vi "Taller3.vi"(10 "U_OUT":dbl min=0.0 max=1.0 step=0.01, 11 "U_IN":dbl min=0.0 max=1.0 step=0.01) -> (0 "Numeric":dbl, 1 "Tank":dbl(slide) scale=0.0..3.3)   [LabVIEW 2024]
panel:
  in  "?":enum16{""}(ring)
  in  "Stop Button":bool
  in  "Alpha":dbl
  in  "A":dbl
  in  "K_OUT":dbl
  in  "DT":dbl
  in  "H_T":dbl
  in  "K_IN":dbl
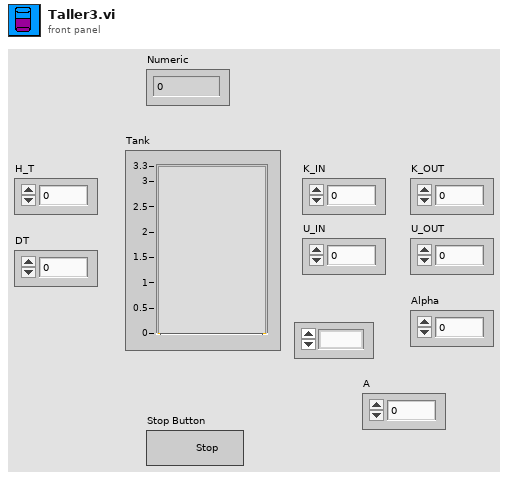
[diagram p1: front panel]
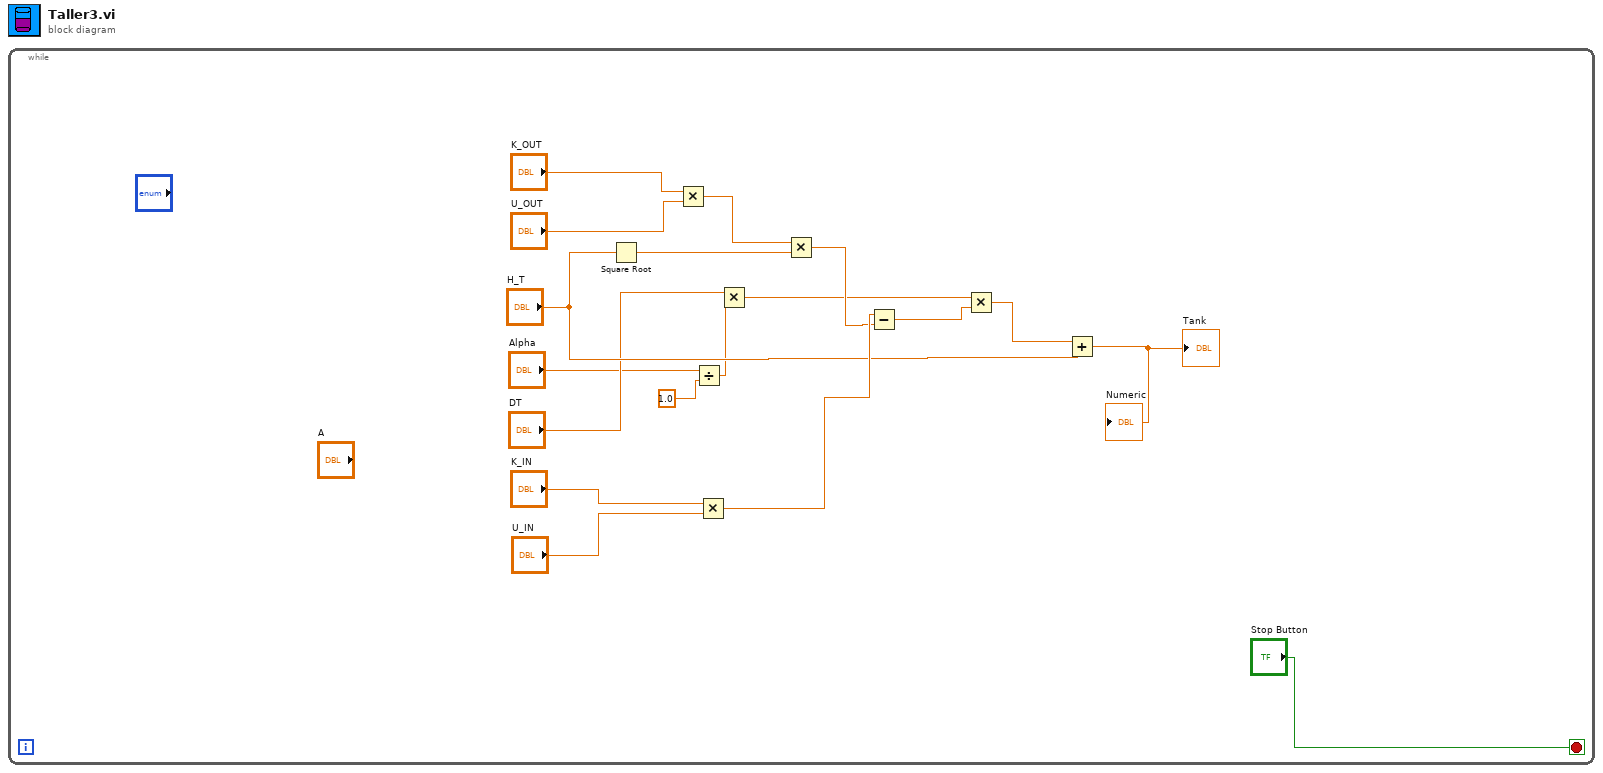
[diagram p0: block diagram]
diagram:
  n1 = while {
    stop <- "Stop Button" stop-if-true
    n2 = Square Root(x="H_T") -> (sqrt(x)=w13:dbl)
    n3 = Multiply(x="K_OUT", y="U_OUT") -> (x*y=w14:dbl)
    n4 = Divide(x="Alpha", y=1.0) -> (x/y=w2:dbl)
    n5 = Multiply(x="K_IN", y="U_IN") -> (x*y=w11:dbl)
    n6 = Multiply(x="DT", y=w2) -> (x*y=w5:dbl)
    n7 = Multiply(x=w14, y=w13) -> (x*y=w10:dbl)
    n8 = Subtract(x=w11, y=w10) -> (x-y=w12:dbl)
    n9 = Multiply(x=w5, y=w12) -> (x*y=w9:dbl)
    n10 = Add(x=w9, y="H_T") -> (x+y=→"Tank" →"Numeric":dbl)
  }
